vi "Check Board Power.vi"() -> (0 "Error Out":errorcluster)   [LabVIEW 2019]
uses:
  <vilib>/regexp/Match Regular Expression.xnode
  <vilib>/myRIO/Instrument Drivers/Utilities/Utilities.lvlib
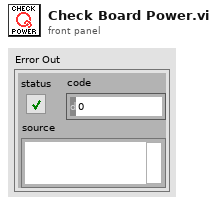
[diagram p1: front panel]
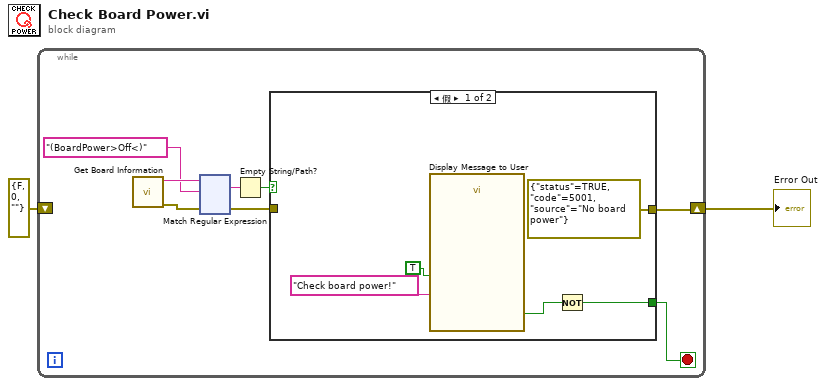
[diagram p0: block diagram]
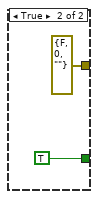
[diagram p2: hidden frame]
diagram:
  n1 = while {
    shift-right: [w4] -> w2
    shift-left: errorcluster {"status"=FALSE, "code"=0, "source"=""} ("error out") -> [_]
    stop <- w3 stop-if-true
    n2 = call <vilib>:"Get Board Information.vi"() -> ("error out"=w8:errorcluster, "Board Information"=w10:string)  [unwired: 10 in]
    n3 = xnode "Match Regular Expression"("input string"=w10, "regular expression"="(BoardPower>Off<)", "error in"=w8) -> ("whole match"=w7:string, "error out"=w6:errorcluster)  [unwired: 3 in, 3 out]
    n4 = Empty String/Path?(string/path=w7) -> (empty?=w5:bool)
    n5 = case shown="假" w5 {
      tunnel: w6 -> [_ _]
      tunnel: [errorcluster {"status"=TRUE, "code"=5001, "source"="No board power"} ("error out") errorcluster {"status"=FALSE, "code"=0, "source"=""} ("error out")] -> w4
      tunnel: [w12 TRUE] -> w3
      frame False {
        n6 = call "Display Message to User"("Enable"=TRUE, "Message"="Check board power!") -> ("OK"=w13:bool)  [unwired: 8 in, 1 out]
        n7 = Not(x=w13) -> (.not. x?=w12:bool)
      }
      frame True {
      }
    }
  }
  "Error Out" <- w2
